vi "SHIFT_DN.vi"(10 "argv":string[](array[string]), 11 "args":u8) -> ()   [LabVIEW 2011]
uses:
  drivetrain/gear_shift_state.ctl
  drivetrain/drivetrain_globals.vi
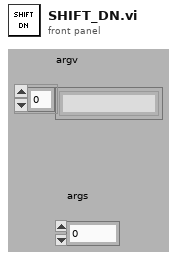
[diagram p1: front panel]
types:
  T1 = typedef "gear_shift_state.ctl" = enum16{"low", "high"}
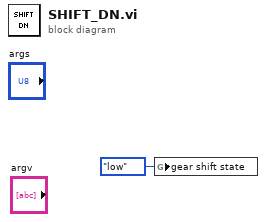
[diagram p0: block diagram]
diagram:
  n1 = global write "drivetrain_globals.vi" "gear shift state"(gear_shift_state."low" ("gear shift state")) -> ()
